vi "Queue_test.vi"() -> ()   [LabVIEW 2021]
panel:
  in  "stop":bool
  in  "Generate":bool
  out "Generate Numbver":dbl
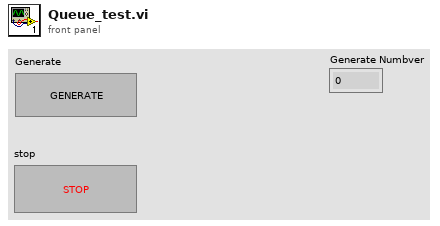
[diagram p1: front panel]
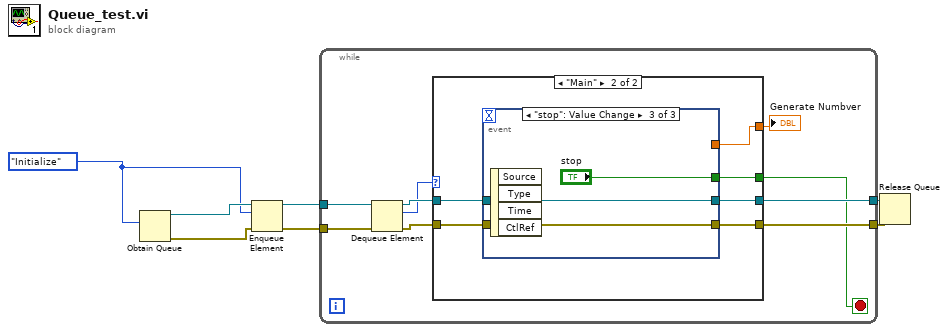
[diagram p0: block diagram]
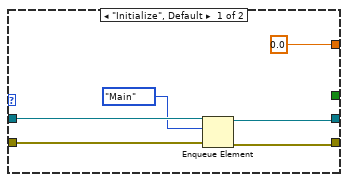
[diagram p2: hidden frame]
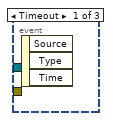
[diagram p3: hidden frame]
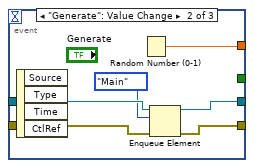
[diagram p4: hidden frame]
diagram:
  w1 = enum16{"Initialize", "Close", "Main"}."Initialize"
  n1 = Obtain Queue(element data type=w1) -> (queue out=w6:refnum<queue>, error out=w7:errorcluster)  [unwired: 4 in, 1 out]
  n2 = Enqueue Element(queue=w6, element=w1, error in (no error)=w7) -> (queue out=w5:refnum<queue>, error out=w4:errorcluster)  [unwired: 1 in, 1 out]
  n3 = while {
    tunnel: w5 -> [w16]
    tunnel: w4 -> [w15]
    tunnel: [w12] -> w3
    tunnel: [w11] -> w2
    stop <- w8 stop-if-true
    n4 = Dequeue Element(queue=w16, error in (no error)=w15) -> (queue out=w14:refnum<queue>, element=w10:enum16{"Initialize", "Close", "Main"}, error out=w13:errorcluster)  [unwired: 1 in, 1 out]
    n5 = case shown="\"Main\"" w10 {
      tunnel: w14 -> [w22 w28]
      tunnel: w13 -> [w21 w27]
      tunnel: [w19 w26] -> w12
      tunnel: [w18 w25] -> w11
      tunnel: [0.0 ("Generate Numbver") w24] -> w9
      tunnel: [_ w23] -> w8
      frame "Initialize", Default {
        n6 = Enqueue Element(queue=w22, element=enum16{"Initialize", "Close", "Main"}."Main", error in (no error)=w21) -> (queue out=w19:refnum<queue>, error out=w18:errorcluster)  [unwired: 1 in, 1 out]
      }
      frame "Main" {
        n7 = event shown="[2] \"stop\": Value Change" {
          selector: _ -> [_ _ _]
          dyn-events: _ -> [_ _ _]
          timeout: _ -> [_ _ _]
          tunnel: w28 -> [_ w33 w37]
          tunnel: w27 -> [_ w32 w36]
          tunnel: [_ w31 w37] -> w26
          tunnel: [_ w30 w36] -> w25
          tunnel: [_ w34 _] -> w24
          tunnel: [_ _ "stop"] -> w23
          event Timeout {
            n8 = event-data() -> ()  [unwired: 1 in, 3 out]
          }
          event "Generate": Value Change {
            n9 = event-data() -> ()  [unwired: 1 in, 4 out]
            n10 = Random Number (0-1)() -> (number: 0 to 1=w34:dbl)
            n11 = Enqueue Element(queue=w33, element=enum16{"Initialize", "Close", "Main"}."Main", error in (no error)=w32) -> (queue out=w31:refnum<queue>, error out=w30:errorcluster)  [unwired: 1 in, 1 out]
          }
          event "stop": Value Change {
            n12 = event-data() -> ()  [unwired: 1 in, 4 out]
          }
        }
      }
    }
    "Generate Numbver" <- w9
  }
  n13 = Release Queue(queue=w3, error in (no error)=w2) -> ()  [unwired: 1 in, 3 out]
